vi "CreateCommunication.vi"(8 "error in (no error)":errorcluster) -> (0 "error out":errorcluster, 3 "Message Queues":T1)   [LabVIEW 2017, in "Client.lvlib" / "CommsFrameWork.lvlib"]
doc: "Creates all Queues and User Events and stores them in References Cluster."
uses:
  CommsFrameWork.lvlib
  TypeDefs/CommReferences.ctl
  TypeDefs/MessageCluster.ctl
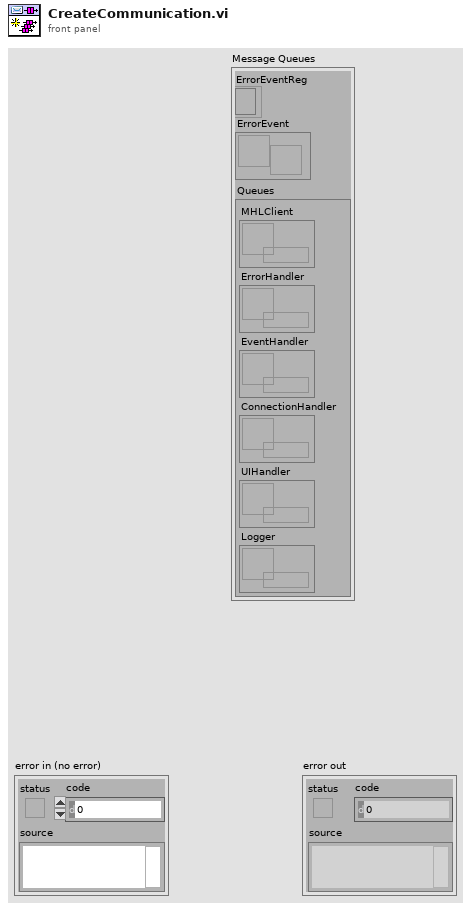
[diagram p1: front panel]
types:
  T1 = typedef "Client.lvlib/CommsFrameWork.lvlib/CommReferences.ctl" = cluster{"ErrorEventReg":refnum<event-registration>, "ErrorEvent":refnum<user-event>, "Queues":cluster{"MHLClient":refnum<queue>, "ErrorHandler":refnum<queue>, "EventHandler":refnum<queue>, "ConnectionHandler":refnum<queue>, "UIHandler":refnum<queue>, "Logger":refnum<queue>}}
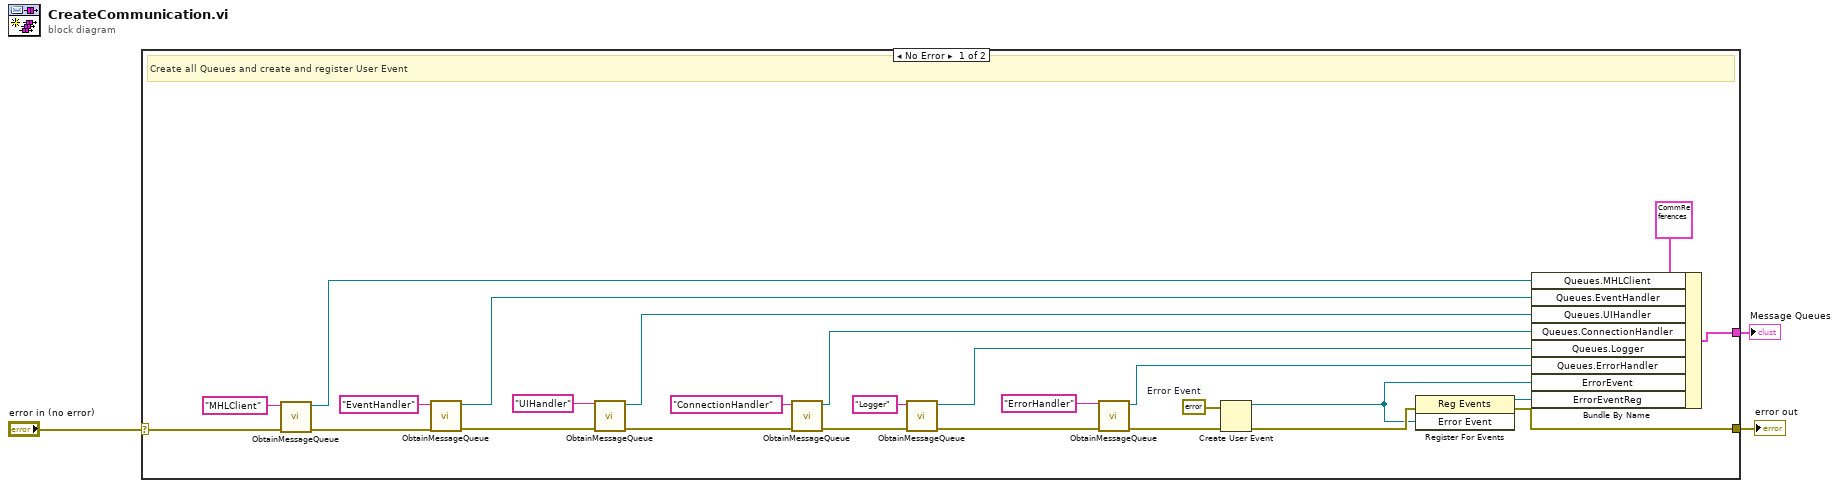
[diagram p0: block diagram]
diagram:
  n1 = case shown="No Error" "error in (no error)" {
    selector: "error in (no error)" -> [w28 w30]
    tunnel: [w6 w30] -> w3
    tunnel: [w29 _] -> w1
    frame No Error {
      w8 = errorcluster {"status"=FALSE, "code"=0, "source"=""}  # Error Event
      # "Create all Queues and create and register User Event"
      n2 = call "ObtainMessageQueue.vi"("error in (no error)"=w28, "Name"="MHLClient") -> ("error out"=w26:errorcluster, "Message Queue"=w17:refnum<queue>)  [unwired: 8 in]
      n3 = call "ObtainMessageQueue.vi"("error in (no error)"=w26, "Name"="EventHandler") -> ("error out"=w25:errorcluster, "Message Queue"=w16:refnum<queue>)  [unwired: 8 in]
      n4 = call "ObtainMessageQueue.vi"("error in (no error)"=w25, "Name"="UIHandler") -> ("error out"=w24:errorcluster, "Message Queue"=w15:refnum<queue>)  [unwired: 8 in]
      n5 = call "ObtainMessageQueue.vi"("error in (no error)"=w24, "Name"="ConnectionHandler") -> ("error out"=w19:errorcluster, "Message Queue"=w14:refnum<queue>)  [unwired: 8 in]
      n6 = call "ObtainMessageQueue.vi"("error in (no error)"=w19, "Name"="Logger") -> ("error out"=w12:errorcluster, "Message Queue"=w13:refnum<queue>)  [unwired: 8 in]
      n7 = call "ObtainMessageQueue.vi"("error in (no error)"=w12, "Name"="ErrorHandler") -> ("error out"=w9:errorcluster, "Message Queue"=w10:refnum<queue>)  [unwired: 8 in]
      n8 = Create User Event(user event datatype=w8, error in=w9) -> (user event=w4:refnum<user-event>, error out=w7:errorcluster)
      n9 = register-events(error in=w7, w4) -> (reference out=w5:refnum<event-registration>, error out=w6:errorcluster)  [unwired: 1 in]
      n10 = Bundle By Name(cluster=T1 {"ErrorEventReg"=refnum, "ErrorEvent"=refnum, "Queues"={"MHLClient"=refnum, "ErrorHandler"=refnum, "EventHandler"=refnum, "ConnectionHandler"=refnum, "UIHandler"=refnum, "Logger"=refnum}} ("Message Queues"), "Queues.MHLClient"=w17, "Queues.EventHandler"=w16, "Queues.UIHandler"=w15, "Queues.ConnectionHandler"=w14, "Queues.Logger"=w13, "Queues.ErrorHandler"=w10, "ErrorEvent"=w4, "ErrorEventReg"=w5) -> (w29:T1)
    }
    frame Error {
    }
  }
  "error out" <- w3
  "Message Queues" <- w1
